vi "Random Number (Range) U64.vi"(10 "lower bound (0)":u64, 11 "upper bound (100)":u64=100) -> (3 "number":u64)   [LabVIEW 2020]
doc: "Generates a random value from a specified range. Wire data to the <B>upper bound</B> or <B>lower bound</B> input to determine the polymorphic instance to use or manually select the instance."
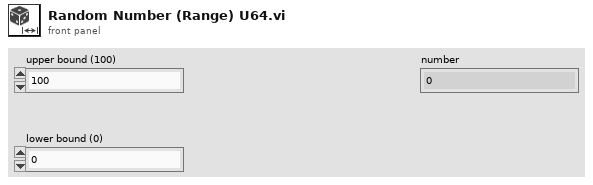
[diagram p1: front panel]
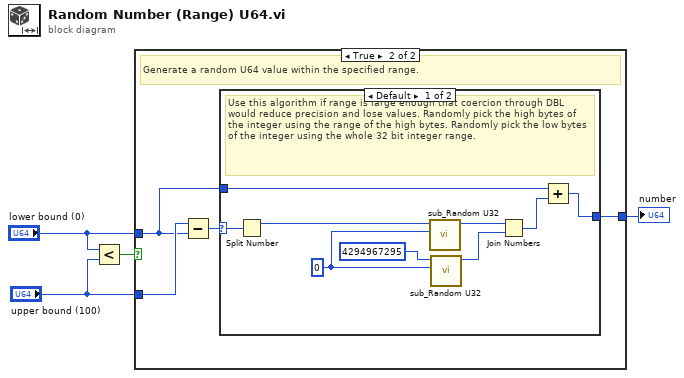
[diagram p0: block diagram]
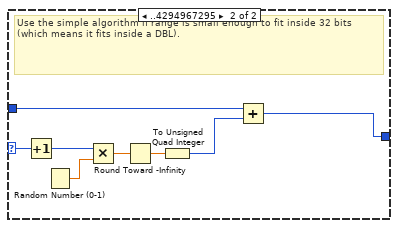
[diagram p3: hidden frame]
diagram:
  n1 = Less?(x="lower bound (0)", y="upper bound (100)") -> (x < y?=w4:bool)
  n2 = case shown="True" w4 {
    tunnel: "lower bound (0)" -> [w5 w7]
    tunnel: "upper bound (100)" -> [_ w9]
    tunnel: [w5 w6] -> w1
    frame False {
      # "If bounds are reversed, always return the lower bound."
    }
    frame True {
      # "Generate a random U64 value within the specified range."
      n3 = Subtract(x=w9, y=w7) -> (x-y=w8:u64)
      n4 = case shown="Default" w8 {
        selector: w8 -> [w18 w24]
        tunnel: w7 -> [w16 w26]
        tunnel: [w15 w25] -> w6
        frame Default {
          w13 = u32 0 ("lower bound")
          # "Use this algorithm if range is large enough that coercion through DBL would reduce precision and lose values. Randomly pick the high bytes of the integer using the range of the high bytes. Randomly pick the low bytes of the integer using the whole 32 bit integer range."
          n5 = Split Number(x=w18) -> (hi(x)=w14:u32)  [unwired: 1 out]
          n6 = call <vilib>:"sub_Random U32.vi"("lower bound"=w13, "upper bound"=w14) -> ("number"=w10:u32)  [unwired: 9 in]
          n7 = call <vilib>:"sub_Random U32.vi"("lower bound"=w13, "upper bound"=u32 4294967295) -> ("number"=w11:u32)  [unwired: 9 in]
          n8 = Join Numbers(hi=w10, lo=w11) -> ((hi.lo)=w17:u64)
          n9 = Add(x=w16, y=w17) -> (x+y=w15:u64)
        }
        frame ..4294967295 {
          # "Use the simple algorithm if range is small enough to fit inside 32 bits (which means it fits inside a DBL)."
          n10 = Increment(x=w24) -> (x+1=w23:u64)
          n11 = Random Number (0-1)() -> (number: 0 to 1=w22:dbl)
          n12 = Multiply(x=w23, y=w22) -> (x*y=w21:dbl)
          n13 = Round Toward -Infinity(1:w21) -> (0:w20:dbl)
          n14 = To Unsigned Quad Integer(1:w20) -> (0:w19:u64)
          n15 = Add(x=w26, y=w19) -> (x+y=w25:u64)
        }
      }
    }
  }
  "number" <- w1
